vi "Task Type.vi"(11 "VolatusConfigTask in":refnum<class "VolatusConfigManager.lvclass">) -> (2 "Task Type":string)   [LabVIEW 2020, in "Volatus.lvlib" / "VolatusConfigManager.lvclass"]
uses:
  VolatusConfigManager.lvclass
  VolatusConfigManager.lvclass/VolatusConfigManager.ctl
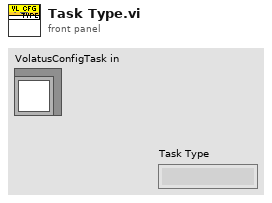
[diagram p1: front panel]
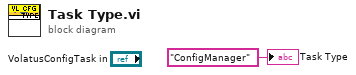
[diagram p0: block diagram]
diagram:
  "Task Type" <- "ConfigManager" ("Task Type")
